vi "Reset Phone.vi"(8 "error in (no error)":errorcluster, 11 "Vision Server in":refnum<class "Vision Server.lvclass">) -> (0 "error out":errorcluster, 3 "Vision Server out":refnum<class "Vision Server.lvclass">)   [LabVIEW 2016, in "Vision Server.lvclass"]
uses:
  Vision Server.lvclass
  Vision Server.lvclass/Vision Server.ctl
  AdbBridge/Adb Bridge.lvclass
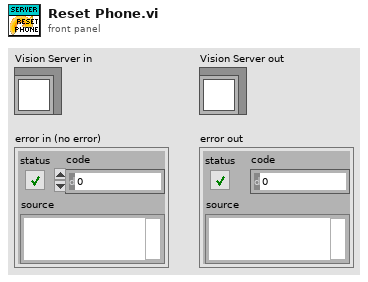
[diagram p1: front panel]
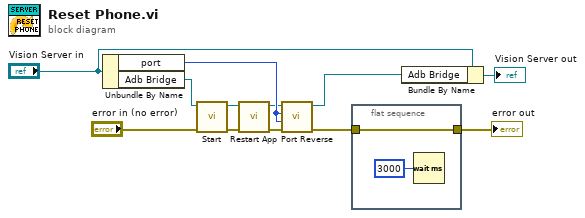
[diagram p0: block diagram]
diagram:
  n1 = Unbundle By Name("Vision Server in") -> ("port"=w12:u16, "Adb Bridge"=w9:refnum<class "Adb Bridge.lvclass">)
  n2 = call "Start.vi"("error in (no error)"="error in (no error)", "AdbBridge in"=w9) -> ("error out"=w5:errorcluster, "AdbBridge out"=w3:refnum<class "Adb Bridge.lvclass">)  [unwired: 8 in]
  n3 = call "Restart App.vi"("error in (no error)"=w5, "AdbBridge in"=w3) -> ("error out"=w6:errorcluster, "AdbBridge out"=w4:refnum<class "Adb Bridge.lvclass">)  [unwired: 8 in]
  n4 = call "Port Reverse.vi"("error in (no error)"=w6, "remote port"=w12, "local port"=w12, "AdbBridge in"=w4) -> ("error out"=w2:errorcluster, "AdbBridge out"=w11:refnum<class "Adb Bridge.lvclass">)  [unwired: 6 in]
  n5 = flat-sequence {
    tunnel: w2 -> [w14]
    tunnel: [w14] -> w1
    frame #0 {
      n6 = Wait (ms)(milliseconds to wait=u32 3000) -> ()  [unwired: 1 out]
    }
  }
  n7 = Bundle By Name(cluster="Vision Server in", "Adb Bridge"=w11) -> (→"Vision Server out":refnum<class "Vision Server.lvclass">)
  "error out" <- w1
